vi "LS One Hour Data Loop.vi"(11 "FPGA OneHour Ref":T1) -> ()   [LabVIEW 2019]
uses:
  <vilib>/rvi/interface/nirviReadWriteControl/nirviReadWriteControl.xnode
  <vilib>/rvi/interface/nirviMethod/nirviMethod.xnode
  <vilib>/FPGAPlugInAG/sbRIO-9626/niLvFpga_ReadFifo_sbRIO-9626.vi
  <vilib>/rvi/errors/niLvFpgaMergeErrorWithErrorCode.vi
  FPGA Bitfiles/LSDurabilityMain_Alternate.lvbitx
  Controls/FPGA_OneHour_Reference.ctl
  NiFpgaLv.dll
  <vilib>/Utility/error.llb/Error Cluster From Error Code.vi
  <vilib>/rvi/errors/niLvFpgaAdjustHostInterfaceError.vi
panel:
  in  "LoopWait(ms)":u32=100
  in  "Sections":i32=100
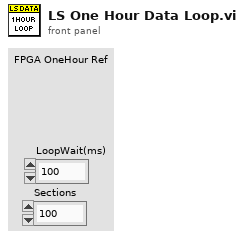
[diagram p1: front panel]
types:
  T1 = typedef "FPGA_OneHour_Reference.ctl" = refnum<k20>
  T2 = cluster{"FPGA OneHour Ref":T1, "Time":dbl, "PtsTaken":i32, "Pts/File":i32, "10AveWait":u32, "Stored Filepath":path, "FileIndex":i32, "FilesUsed":i32}
  T3 = enum16{"open", "replace", "create", "open or create", "replace or create", "replace or create with confirmation"}
  T4 = cluster{"Running?":bool, "Profile Record":bool, "RecordInterval":i32, "RecordDuration":i32, "RecordFreq":i32, "Data Filepath":path, "Hr Record":bool, "Serial Numbers":string[]}
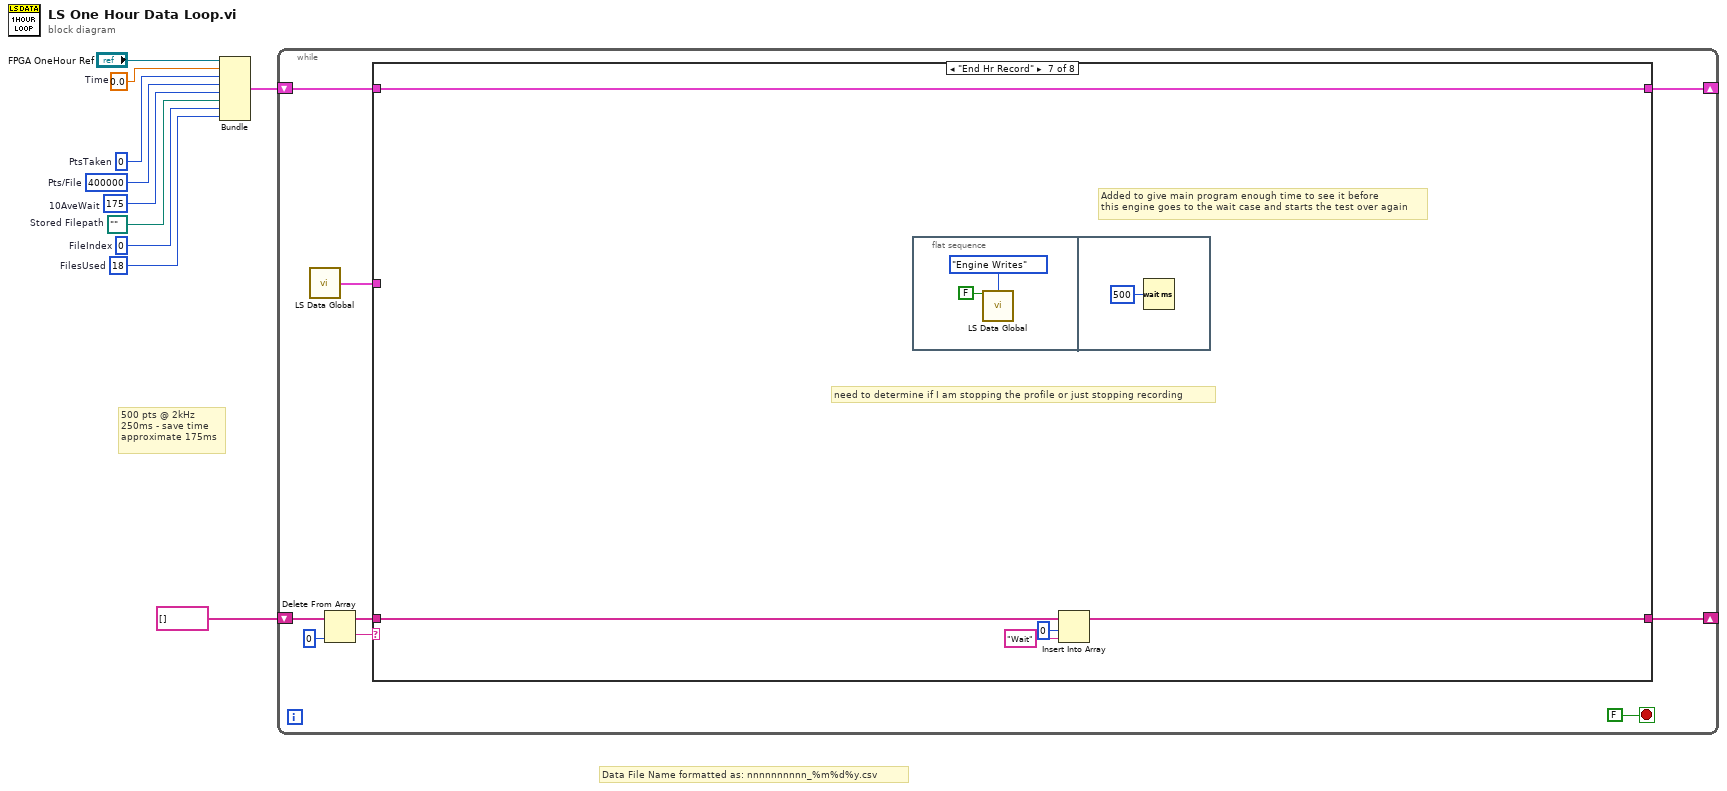
[diagram p0: block diagram]
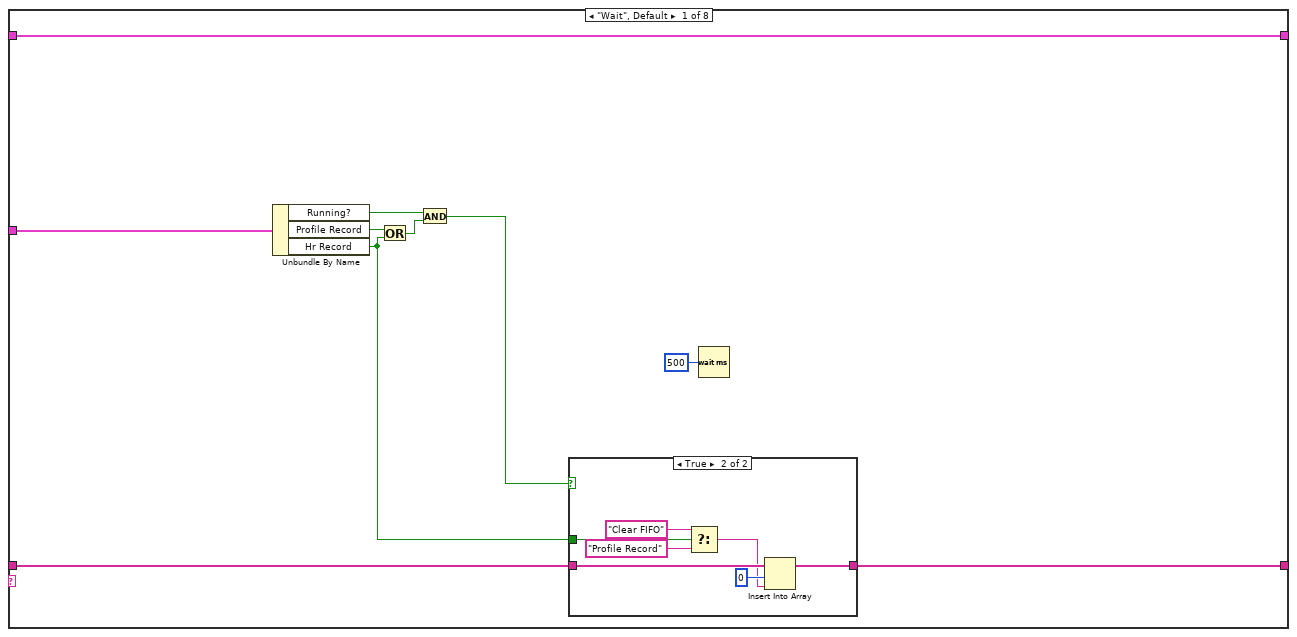
[diagram p2: hidden frame]
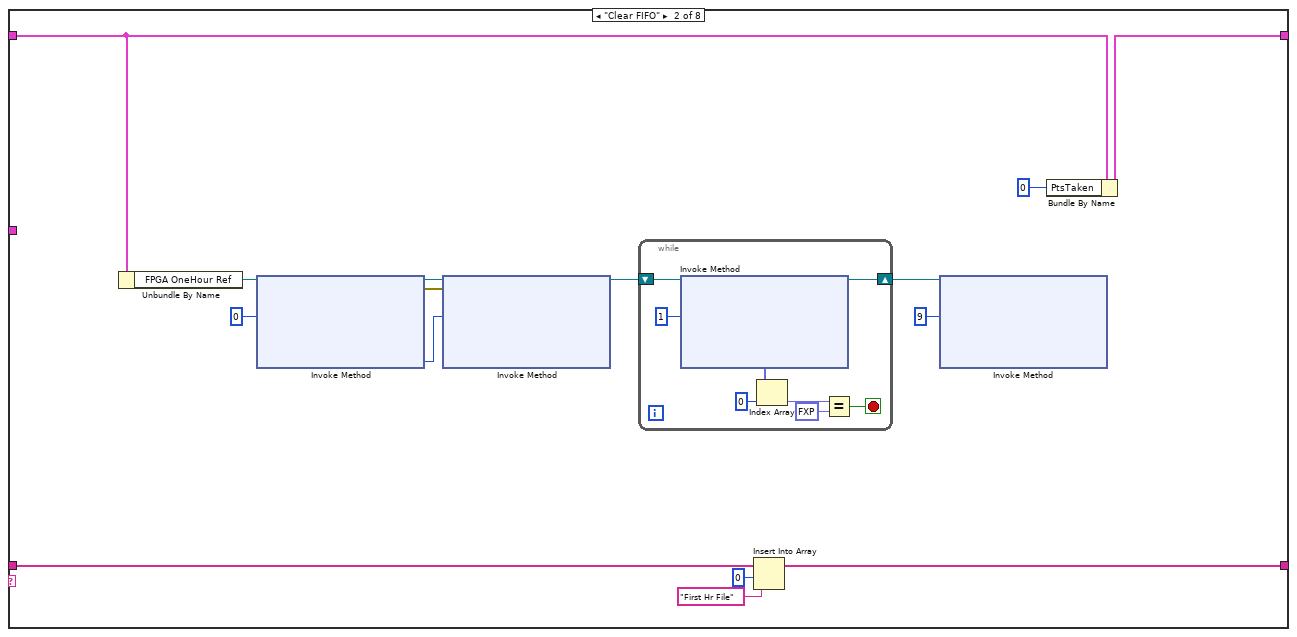
[diagram p4: hidden frame]
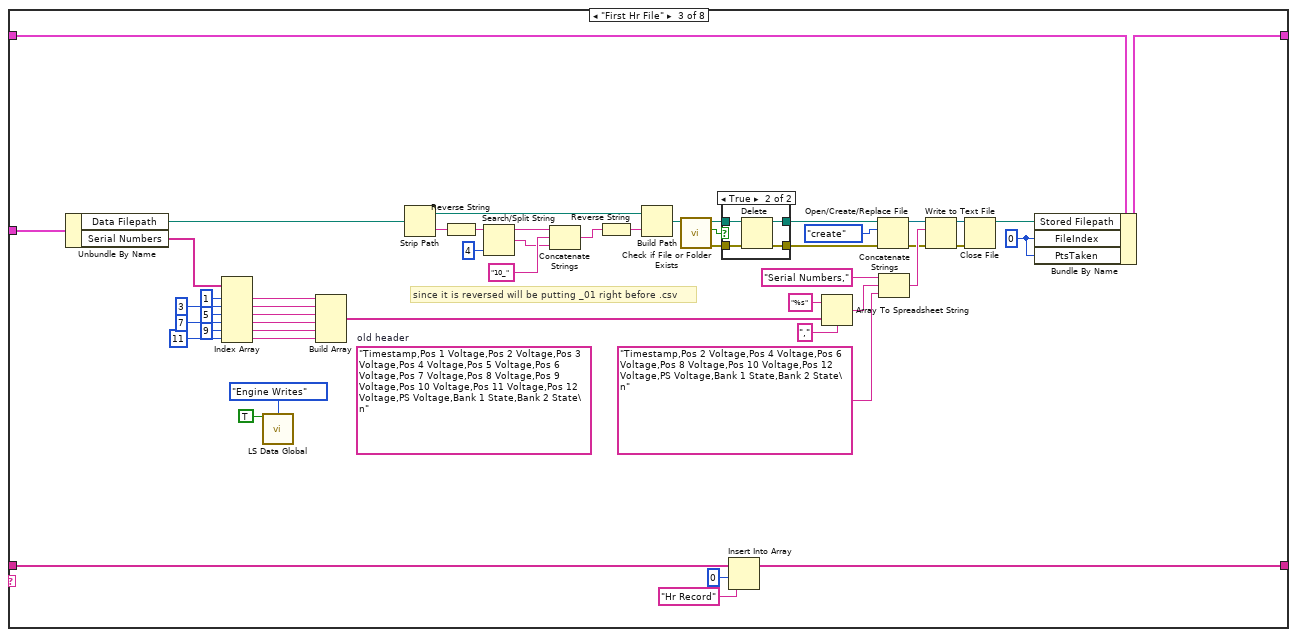
[diagram p5: hidden frame]
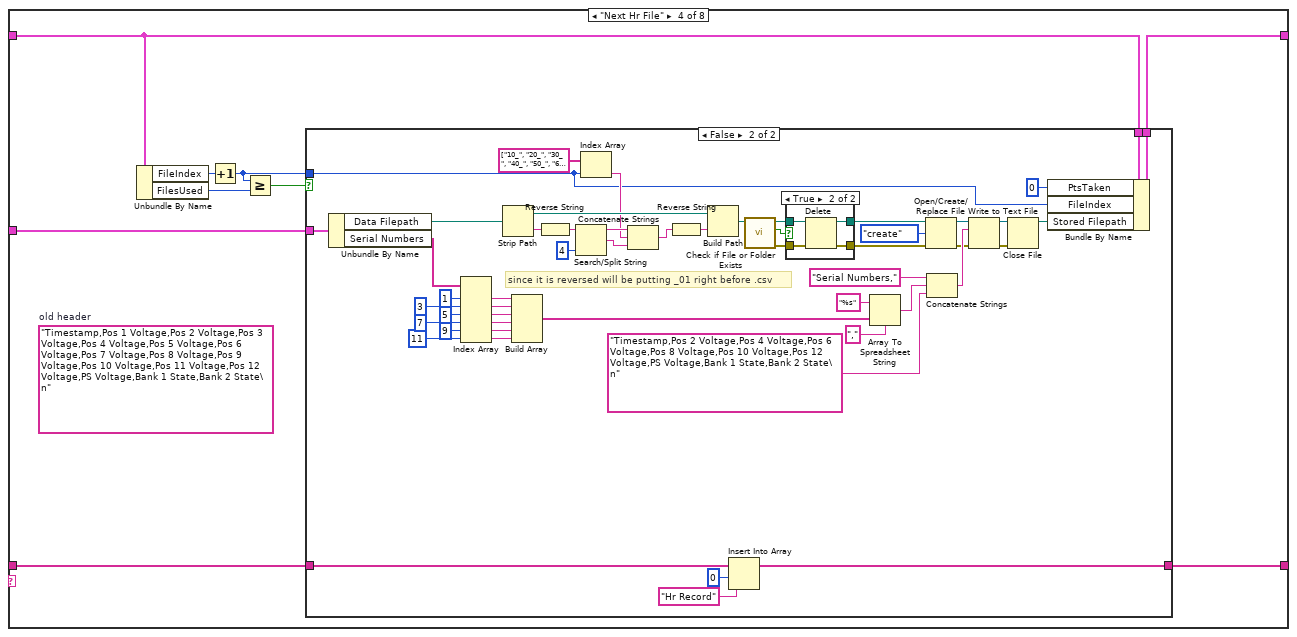
[diagram p7: hidden frame]
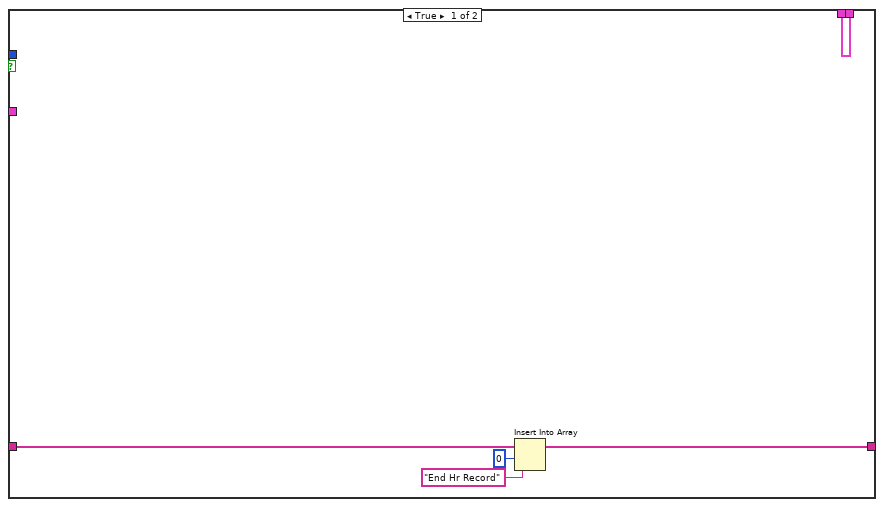
[diagram p8: hidden frame]
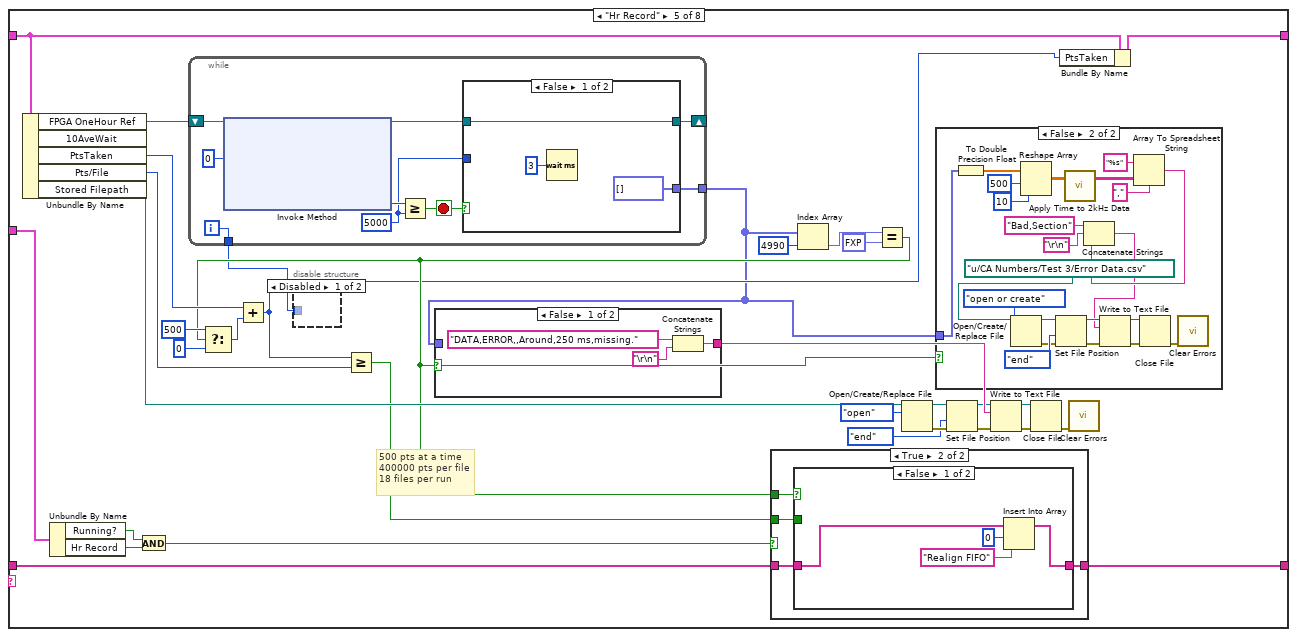
[diagram p10: hidden frame]
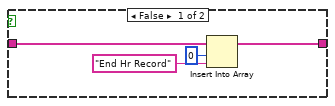
[diagram p13: hidden frame]
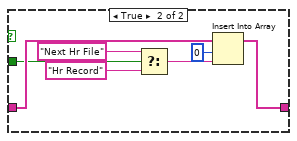
[diagram p14: hidden frame]
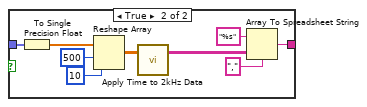
[diagram p15: hidden frame]
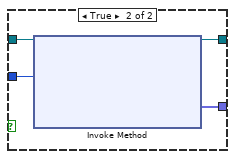
[diagram p16: hidden frame]
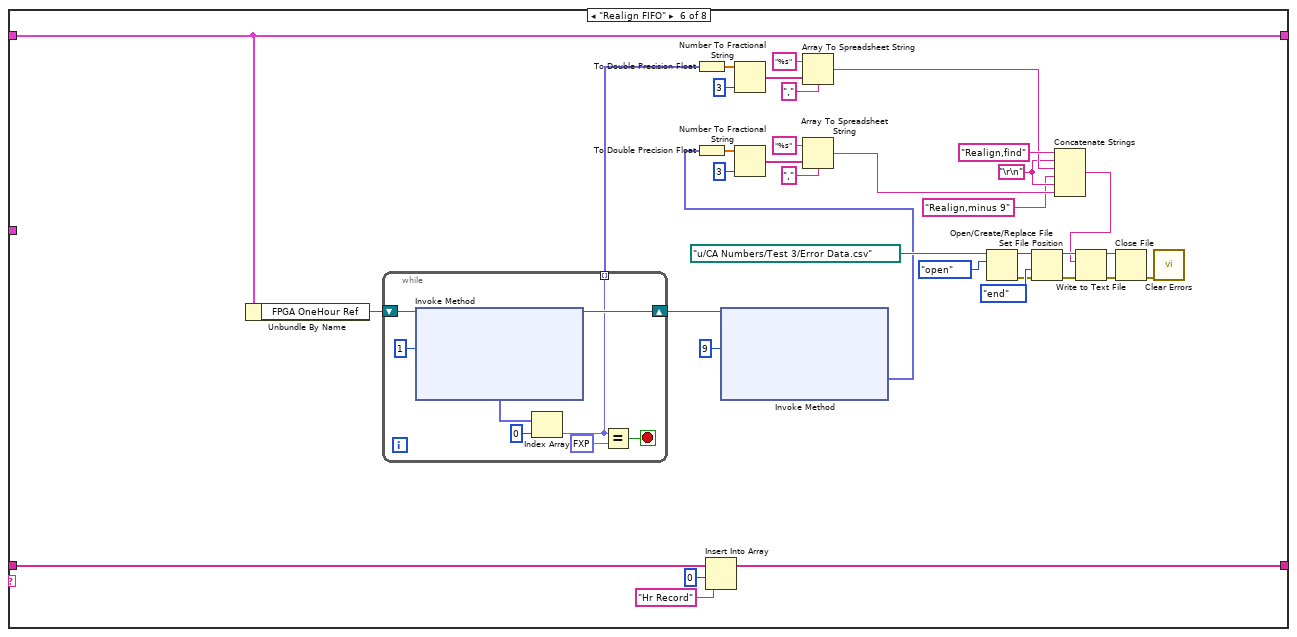
[diagram p17: hidden frame]
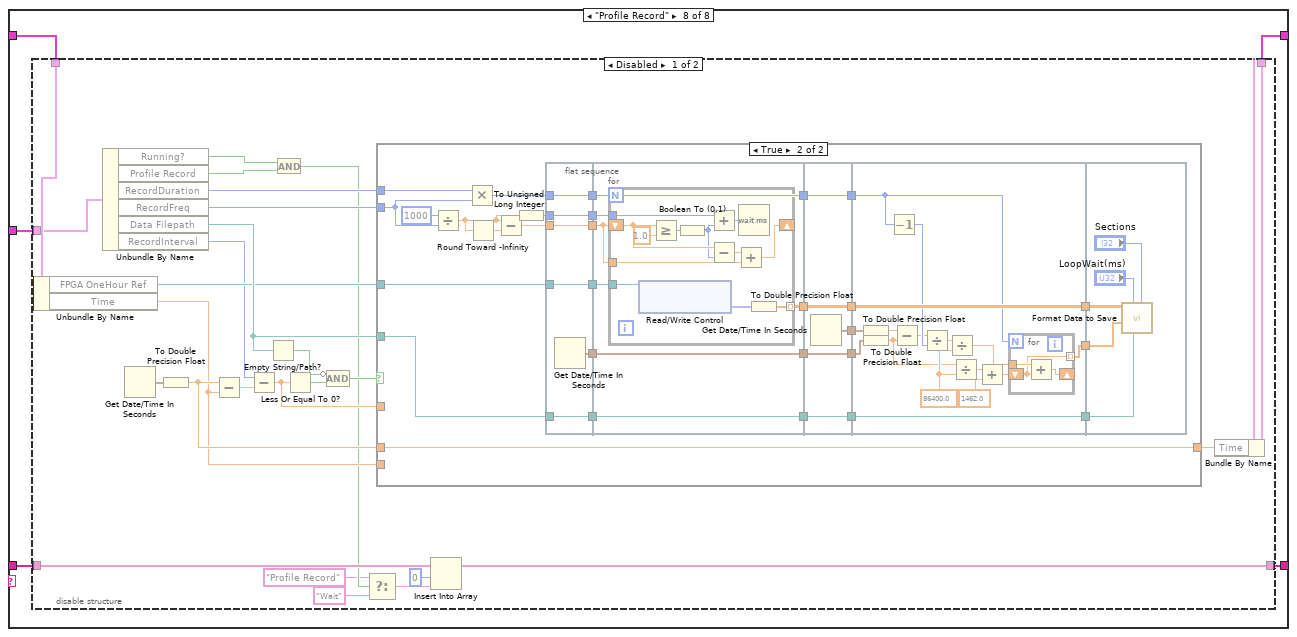
[diagram p18: hidden frame]
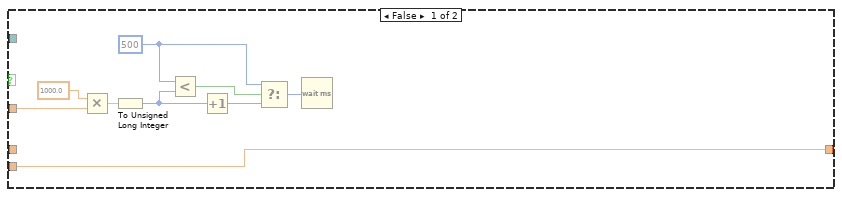
[diagram p19: hidden frame]
diagram:
  w1 = 18  # FilesUsed
  w2 = 400000  # Pts/File
  w4 = 0  # FileIndex
  w5 = path ""  # Stored Filepath
  w6 = u32 175  # 10AveWait
  w7 = 0  # PtsTaken
  w10 = 0.0  # Time
  # "500 pts @ 2kHz\n250ms - save time\napproximate 175ms"
  # "Data File Name formatted as: nnnnnnnnnn_%m%d%y.csv"
  n1 = Bundle("FPGA OneHour Ref"="FPGA OneHour Ref", "Time"=w10, "PtsTaken"=w7, "Pts/File"=w2, "10AveWait"=w6, "Stored Filepath"=w5, "FileIndex"=w4, "FilesUsed"=w1) -> (w9:T2)  [unwired: 1 in]
  n2 = while {
    shift-right: [w17] -> _
    shift-left: w9 -> [w18]
    shift-right: [w14] -> _
    shift-left: string[] [] -> [w16]
    stop <- FALSE stop-if-true
    n3 = call "LS Data Global.vi"() -> ("LS Cluster Out"=w15:T4)  [unwired: 12 in, 3 out]
    n4 = Delete From Array(array=w16, index=0) -> (deleted portion=w12:string, array with subset deleted=w11:string[])  [unwired: 1 in]
    n5 = case shown="\"End Hr Record\"" w12 {
      tunnel: w11 -> [w26 w47 w99 w119 w204 w322 w340 w346]
      tunnel: [w25 w45 w98 w125 w205 w321 w339 w345] -> w14
      tunnel: w15 -> [w27 _ w111 w127 w221 _ _ w347]
      tunnel: w18 -> [w24 w43 w112 w124 w199 w325 w341 w349]
      tunnel: [w24 w42 w110 w126 w198 w325 w341 w348] -> w17
      frame "Wait", Default {
        n6 = Unbundle By Name(w27) -> ("Running?"=w28:bool, "Profile Record"=w23:bool, "Hr Record"=w21:bool)
        n7 = Or(x=w23, y=w21) -> (x .or. y?=w22:bool)
        n8 = And(x=w28, y=w22) -> (x .and. y?=w20:bool)
        n9 = case shown="True" w20 {
          tunnel: w26 -> [w30 w37]
          tunnel: [w30 w36] -> w25
          tunnel: w21 -> [_ w34]
          frame False {
          }
          frame True {
            n10 = Select(t="Clear FIFO" ("new element/subarray"), s=w34, f="Profile Record" ("new element/subarray")) -> (s? t:f=w32:string)
            n11 = Insert Into Array(array=w37, index=0, new element=w32) -> (w36:string[])
          }
        }
        n12 = Wait (ms)(milliseconds to wait=u32 500) -> ()  [unwired: 1 out]
      }
      frame "Clear FIFO" {
        n13 = Unbundle By Name(w43) -> ("FPGA OneHour Ref"=w52:T1)
        n14 = xnode "Invoke Method"("FPGA VI Reference In"=w52, "Number of Elements"=u32 0) -> ("FPGA VI Reference Out"=w51:T1, "error out"=w50:errorcluster, "Elements Remaining"=w48:u32)  [unwired: 2 in, 1 out]
        n15 = xnode "Invoke Method"("FPGA VI Reference In"=w51, "error in"=w50, "Number of Elements"=w48) -> ("FPGA VI Reference Out"=w40:T1)  [unwired: 1 in, 3 out]
        n16 = while {
          shift-right: [w59] -> w38
          shift-left: w40 -> [w60]
          stop <- w53 stop-if-true
          n17 = xnode "Invoke Method"("FPGA VI Reference In"=w60, "Number of Elements"=u32 1) -> ("FPGA VI Reference Out"=w59:T1, "Data"=w57:fxp<+/-,18,5>[])  [unwired: 2 in, 2 out]
          n18 = Index Array(array=w57, index=0) -> (element=w55:fxp<+/-,18,5>)
          n19 = Equal?(x=w55, y=fxp<+/-,18,5> -15.0 ("lower limit")) -> (x = y?=w53:bool)
        }
        n20 = Insert Into Array(array=w47, index=0, new element="First Hr File" ("new element/subarray")) -> (w45:string[])
        n21 = xnode "Invoke Method"("FPGA VI Reference In"=w38, "Number of Elements"=u32 9) -> ()  [unwired: 2 in, 4 out]
        n22 = Bundle By Name(cluster=w43, "PtsTaken"=0) -> (w42:T2)
      }
      frame "First Hr File" {
        (unwired) "Timestamp,Pos 1 Voltage,Pos 2 Voltage,Pos 3 Voltage,Pos 4 Voltage,Pos 5 Voltage,Pos 6 Voltage,Pos 7 Voltage,Pos 8 Voltage,Pos 9 Voltage,Pos 10 Voltage,Pos 11 Voltage,Pos 12 Voltage,PS Voltage,Bank 1 State,Bank 2 State\n"  # old header
        w77 = 0 ("FileIndex")
        # "since it is reversed will be putting _01 right before .csv"
        n23 = Unbundle By Name(w111) -> ("Data Filepath"=w109:path, "Serial Numbers"=w62:string[])
        n24 = Index Array(array=w62, index #1=1 ("index"), index #2=3 ("index"), index #3=5 ("index"), index #4=7 ("index"), index #5=9 ("index"), index #6=11 ("index")) -> (element #1=w68:string, element #2=w67:string, element #3=w66:string, element #4=w65:string, element #5=w63:string, element #6=w64:string)
        n25 = call "LS Data Global.vi"("Recording In"=TRUE, "Mode"=enum16{"Read", "Engine Writes", "Main Writes"}."Engine Writes") -> ()  [unwired: 10 in, 4 out]
        n26 = Build Array(w68, w67, w66, w65, w63, w64) -> (w61:string[])
        n27 = Strip Path(path=w109) -> (stripped path=w108:path, name=w107:string)
        n28 = Reverse String(1:w107) -> (0:w105:string)
        n29 = Search/Split String(string=w105, offset (0)=4) -> (substring before match=w103:string, match + rest of string=w100:string)  [unwired: 1 in, 1 out]
        n30 = Concatenate Strings(w103, "10_", w100) -> (w102:string)
        n31 = Reverse String(1:w102) -> (0:w106:string)
        n32 = Build Path(base path=w108, name or relative path=w106) -> (appended path=w95:path)
        n33 = call <vilib>:"Check if File or Folder Exists.vi"("path"=w95) -> ("error out"=w80:errorcluster, "file or folder exists?"=w94:bool, "dup path"=w93:path)  [unwired: 8 in]
        n34 = case shown="True" w94 {
          tunnel: w93 -> [w114 w118]
          tunnel: [w114 w117] -> w82
          tunnel: w80 -> [w113 w116]
          tunnel: [w113 w115] -> w79
          frame False {
          }
          frame True {
            n35 = Delete(path (use dialog)=w118, error in=w116) -> (deleted path=w117:path, error out=w115:errorcluster)  [unwired: 3 in, 1 out]
          }
        }
        n36 = Insert Into Array(array=w99, index=0, new element="Hr Record" ("new element/subarray")) -> (w98:string[])
        n37 = Array To Spreadsheet String(delimiter (Tab)=",", array=w61, 3:"%s" ("format string")) -> (spreadsheet string=w92:string)
        n38 = Open/Create/Replace File(file path (use dialog)=w82, error in=w79, operation (0:open)=T3."create") -> (refnum out=w86:refnum<file>, error out=w84:errorcluster)  [unwired: 3 in, 1 out]
        n39 = Concatenate Strings("Serial Numbers," ("string"), w92, "Timestamp,Pos 2 Voltage,Pos 4 Voltage,Pos 6 Voltage,Pos 8 Voltage,Pos 10 Voltage,Pos 12 Voltage,PS Voltage,Bank 1 State,Bank 2 State\n") -> (w89:string)
        n40 = Write to Text File(file (use dialog)=w86, text=w89, error in=w84) -> (refnum out=w87:refnum<file>, error out=w85:errorcluster)  [unwired: 1 in, 1 out]
        n41 = Close File(refnum=w87, error in=w85) -> (path=w81:path)  [unwired: 1 out]
        n42 = Bundle By Name(cluster=w112, "Stored Filepath"=w81, "FileIndex"=w77, "PtsTaken"=w77) -> (w110:T2)
      }
      frame "Next Hr File" {
        (unwired) "Timestamp,Pos 1 Voltage,Pos 2 Voltage,Pos 3 Voltage,Pos 4 Voltage,Pos 5 Voltage,Pos 6 Voltage,Pos 7 Voltage,Pos 8 Voltage,Pos 9 Voltage,Pos 10 Voltage,Pos 11 Voltage,Pos 12 Voltage,PS Voltage,Bank 1 State,Bank 2 State\n"  # old header
        n43 = Unbundle By Name(w124) -> ("FileIndex"=w123:i32, "FilesUsed"=w122:i32)
        n44 = Increment(x=w123) -> (x+1=w121:i32)
        n45 = Greater Or Equal?(x=w121, y=w122) -> (x >= y?=w120:bool)
        n46 = case shown="False" w120 {
          tunnel: w127 -> [_ w184]
          tunnel: [w132 w183] -> w126
          tunnel: [w130 w172] -> w125
          tunnel: w124 -> [w132 w152]
          tunnel: w121 -> [_ w149]
          tunnel: w119 -> [w131 w173]
          frame True {
            n47 = Insert Into Array(array=w131, index=0, new element="End Hr Record" ("new element/subarray")) -> (w130:string[])
          }
          frame False {
            # "since it is reversed will be putting _01 right before .csv"
            n48 = Unbundle By Name(w184) -> ("Data Filepath"=w182:path, "Serial Numbers"=w134:string[])
            n49 = Index Array(array=w134, index #1=1 ("index"), index #2=3 ("index"), index #3=5 ("index"), index #4=7 ("index"), index #5=9 ("index"), index #6=11 ("index")) -> (element #1=w140:string, element #2=w139:string, element #3=w138:string, element #4=w137:string, element #5=w135:string, element #6=w136:string)
            n50 = Strip Path(path=w182) -> (stripped path=w181:path, name=w180:string)
            n51 = Build Array(w140, w139, w138, w137, w135, w136) -> (w133:string[])
            n52 = Reverse String(1:w180) -> (0:w178:string)
            n53 = Search/Split String(string=w178, offset (0)=4) -> (substring before match=w176:string, match + rest of string=w174:string)  [unwired: 1 in, 1 out]
            n54 = Index Array(array=string[] ["10_", "20_", "30_", "40_", "50_", "60_", "70_", "80_", "90_", "01_", "11_", "21_", "31_", "41_", "51_", "61_", "71_", "81_", "91_", "02_", "12_", "22_", "32_", "42_", "52_", "62_", "72_", "82_", "92_", "03_", "13_", "23_"], index=w149) -> (element=w150:string)
            n55 = Concatenate Strings(w176, w150, w174) -> (w175:string)
            n56 = Reverse String(1:w175) -> (0:w179:string)
            n57 = Build Path(base path=w181, name or relative path=w179) -> (appended path=w169:path)
            n58 = Insert Into Array(array=w173, index=0, new element="Hr Record" ("new element/subarray")) -> (w172:string[])
            n59 = call <vilib>:"Check if File or Folder Exists.vi"("path"=w169) -> ("error out"=w154:errorcluster, "file or folder exists?"=w168:bool, "dup path"=w167:path)  [unwired: 8 in]
            n60 = case shown="True" w168 {
              tunnel: w167 -> [w186 w190]
              tunnel: [w186 w189] -> w156
              tunnel: w154 -> [w185 w188]
              tunnel: [w185 w187] -> w153
              frame False {
              }
              frame True {
                n61 = Delete(path (use dialog)=w190, error in=w188) -> (deleted path=w189:path, error out=w187:errorcluster)  [unwired: 3 in, 1 out]
              }
            }
            n62 = Array To Spreadsheet String(delimiter (Tab)=",", array=w133, 3:"%s" ("format string")) -> (spreadsheet string=w166:string)
            n63 = Open/Create/Replace File(file path (use dialog)=w156, error in=w153, operation (0:open)=T3."create") -> (refnum out=w160:refnum<file>, error out=w158:errorcluster)  [unwired: 3 in, 1 out]
            n64 = Concatenate Strings("Serial Numbers," ("string"), w166, "Timestamp,Pos 2 Voltage,Pos 4 Voltage,Pos 6 Voltage,Pos 8 Voltage,Pos 10 Voltage,Pos 12 Voltage,PS Voltage,Bank 1 State,Bank 2 State\n") -> (w163:string)
            n65 = Write to Text File(file (use dialog)=w160, text=w163, error in=w158) -> (refnum out=w161:refnum<file>, error out=w159:errorcluster)  [unwired: 1 in, 1 out]
            n66 = Close File(refnum=w161, error in=w159) -> (path=w155:path)  [unwired: 1 out]
            n67 = Bundle By Name(cluster=w152, "PtsTaken"=0, "FileIndex"=w149, "Stored Filepath"=w155) -> (w183:T2)
          }
        }
      }
      frame "Hr Record" {
        # "500 pts at a time\n400000 pts per file\n18 files per run"
        n68 = Unbundle By Name(w199) -> ("FPGA OneHour Ref"=w193:T1, "PtsTaken"=w203:i32, "Pts/File"=w197:i32, "Stored Filepath"=w210:path)  [unwired: 1 out]
        n69 = Unbundle By Name(w221) -> ("Running?"=w222:bool, "Hr Record"=w223:bool)
        n70 = And(x=w222, y=w223) -> (x .and. y?=w206:bool)
        n71 = while {
          shift-right: [w280] -> _
          shift-left: w193 -> [w283]
          tunnel: [w279] -> w192
          tunnel: [w277] -> w191
          i -> [w277]
          stop <- w278 stop-if-true
          w282 = u32 5000 ("y")
          n72 = xnode "Invoke Method"("FPGA VI Reference In"=w283, "Number of Elements"=u32 0) -> ("FPGA VI Reference Out"=w281:T1, "Elements Remaining"=w284:u32)  [unwired: 2 in, 2 out]
          n73 = Greater Or Equal?(x=w284, y=w282) -> (x >= y?=w278:bool)
          n74 = case shown="False" w278 {
            tunnel: w282 -> [_ w292]
            tunnel: w281 -> [w288 w291]
            tunnel: [w288 w290] -> w280
            tunnel: [fxp<+/-,18,5>[] [] ("Data") w289] -> w279
            frame False {
              n75 = Wait (ms)(milliseconds to wait=u32 3) -> ()  [unwired: 1 out]
            }
            frame True {
              n76 = xnode "Invoke Method"("FPGA VI Reference In"=w291, "Number of Elements"=w292) -> ("FPGA VI Reference Out"=w290:T1, "Data"=w289:fxp<+/-,18,5>[])  [unwired: 2 in, 2 out]
            }
          }
        }
        n77 = disable-structure shown="Disabled" {
          disable-tunnel: w191 -> [_ _]
          frame Disabled {
          }
          frame Enabled {
          }
        }
        n78 = Index Array(array=w192, index=4990) -> (element=w208:fxp<+/-,18,5>)
        n79 = Equal?(x=w208, y=fxp<+/-,18,5> -15.0) -> (x = y?=w195:bool)
        n80 = Select(t=500 ("PtsTaken"), s=w195, f=0 ("PtsTaken")) -> (s? t:f=w200:i32)
        n81 = Add(x=w203, y=w200) -> (x+y=w194:i32)
        n82 = Greater Or Equal?(x=w194, y=w197) -> (x >= y?=w196:bool)
        n83 = case shown="False" w195 {
          tunnel: [w265 w272] -> w213
          tunnel: w192 -> [_ w269]
          frame False {
            n84 = Concatenate Strings("DATA,ERROR,,Around,250 ms,missing." ("string"), "\r\n") -> (w265:string)
          }
          frame True {
            n85 = To Single Precision Float(number=w269) -> (single precision float=w268:sgl[])
            n86 = Reshape Array(w268, 500 ("dimension size"), 10 ("dimension size")) -> (w271:sgl[][])
            n87 = call "Apply Time to 2kHz Data.vi"("Data In"=w271) -> ("Data Out"=w270:string[][])  [unwired: 2 in]
            n88 = Array To Spreadsheet String(delimiter (Tab)=",", array=w270, 3:"%s" ("format string")) -> (spreadsheet string=w272:string)
          }
        }
        n89 = case shown="True" w206 {
          tunnel: w204 -> [w248 w252]
          tunnel: [w247 w251] -> w205
          tunnel: w195 -> [_ w253]
          tunnel: w196 -> [_ w250]
          frame False {
            n90 = Insert Into Array(array=w248, index=0, new element="End Hr Record") -> (w247:string[])
          }
          frame True {
            n91 = case shown="False" w253 {
              tunnel: w252 -> [w257 w264]
              tunnel: [w256 w263] -> w251
              tunnel: w250 -> [_ w261]
              frame False {
                n92 = Insert Into Array(array=w257, index=0, new element="Realign FIFO" ("new element/subarray")) -> (w256:string[])
              }
              frame True {
                n93 = Select(t="Next Hr File", s=w261, f="Hr Record") -> (s? t:f=w260:string)
                n94 = Insert Into Array(array=w264, index=0, new element=w260) -> (w263:string[])
              }
            }
          }
        }
        n95 = Open/Create/Replace File(file path (use dialog)=w210, operation (0:open)=T3."open") -> (refnum out=w216:refnum<file>, error out=w215:errorcluster)  [unwired: 4 in, 1 out]
        n96 = case shown="False" w195 {
          tunnel: w192 -> [_ w240]
          frame True {
          }
          frame False {
            n97 = To Double Precision Float(number=w240) -> (double precision float=w243:dbl[])
            n98 = Open/Create/Replace File(file path (use dialog)=path "u:/CA Numbers/Test 3/Error Data.csv" ("base path"), operation (0:open)=T3."open or create") -> (refnum out=w233:refnum<file>, error out=w234:errorcluster)  [unwired: 4 in, 1 out]
            n99 = Reshape Array(w243, 500 ("dimension size"), 10 ("dimension size")) -> (w239:dbl[][])
            n100 = Set File Position(refnum=w233, from (0:start)=enum16{"start", "end", "current"}."end", error in=w234) -> (refnum out=w236:refnum<file>, error out=w237:errorcluster)  [unwired: 1 in]
            n101 = call "Apply Time to 2kHz Data.vi"("Data In"=w239) -> ("Data Out"=w238:string[][])  [unwired: 2 in]
            n102 = Array To Spreadsheet String(delimiter (Tab)=",", array=w238, 3:"%s" ("format string")) -> (spreadsheet string=w226:string)
            n103 = Concatenate Strings("Bad,Section" ("string"), "\r\n", w226) -> (w225:string)
            n104 = Write to Text File(file (use dialog)=w236, text=w225, error in=w237) -> (refnum out=w230:refnum<file>, error out=w229:errorcluster)  [unwired: 1 in, 1 out]
            n105 = Close File(refnum=w230, error in=w229) -> (error out=w231:errorcluster)  [unwired: 1 out]
            n106 = call <vilib>:"Clear Errors.vi"("error in (no error)"=w231) -> ()  [unwired: 5 in, 2 out]
          }
        }
        n107 = Set File Position(refnum=w216, from (0:start)=enum16{"start", "end", "current"}."end", error in=w215) -> (refnum out=w212:refnum<file>, error out=w211:errorcluster)  [unwired: 1 in]
        n108 = Write to Text File(file (use dialog)=w212, text=w213, error in=w211) -> (refnum out=w219:refnum<file>, error out=w220:errorcluster)  [unwired: 1 in, 1 out]
        n109 = Close File(refnum=w219, error in=w220) -> (error out=w218:errorcluster)  [unwired: 1 out]
        n110 = Bundle By Name(cluster=w199, "PtsTaken"=w194) -> (w198:T2)
        n111 = call <vilib>:"Clear Errors.vi"("error in (no error)"=w218) -> ()  [unwired: 5 in, 2 out]
      }
      frame "Realign FIFO" {
        w301 = "\r\n"
        n112 = Unbundle By Name(w325) -> ("FPGA OneHour Ref"=w328:T1)
        n113 = while {
          shift-right: [w335] -> w326
          shift-left: w328 -> [w336]
          tunnel: [w329] -> w305 mode=indexing
          stop <- w330 stop-if-true
          n114 = xnode "Invoke Method"("FPGA VI Reference In"=w336, "Number of Elements"=u32 1) -> ("FPGA VI Reference Out"=w335:T1, "Data"=w333:fxp<+/-,18,5>[])  [unwired: 2 in, 2 out]
          n115 = Index Array(array=w333, index=0) -> (element=w329:fxp<+/-,18,5>)
          n116 = Equal?(x=w329, y=fxp<+/-,18,5> -15.0 ("lower limit")) -> (x = y?=w330:bool)
        }
        n117 = To Double Precision Float(number=w305) -> (double precision float=w303:dbl[])
        n118 = Insert Into Array(array=w322, index=0, new element="Hr Record" ("new element/subarray")) -> (w321:string[])
        n119 = xnode "Invoke Method"("FPGA VI Reference In"=w326, "Number of Elements"=u32 9) -> ("Data"=w295:fxp<+/-,18,5>[])  [unwired: 2 in, 3 out]
        n120 = To Double Precision Float(number=w295) -> (double precision float=w299:dbl[])
        n121 = Number To Fractional String(number=w303, precision (6)=i16 3) -> (F-format string=w302:string[])  [unwired: 2 in]
        n122 = Number To Fractional String(number=w299, precision (6)=i16 3) -> (F-format string=w300:string[])  [unwired: 2 in]
        n123 = Array To Spreadsheet String(delimiter (Tab)=",", array=w302, 3:"%s" ("format string")) -> (spreadsheet string=w308:string)
        n124 = Array To Spreadsheet String(delimiter (Tab)=",", array=w300, 3:"%s" ("format string")) -> (spreadsheet string=w294:string)
        n125 = Open/Create/Replace File(file path (use dialog)=path "u:/CA Numbers/Test 3/Error Data.csv" ("base path"), operation (0:open)=T3."open") -> (refnum out=w314:refnum<file>, error out=w315:errorcluster)  [unwired: 4 in, 1 out]
        n126 = Set File Position(refnum=w314, from (0:start)=enum16{"start", "end", "current"}."end", error in=w315) -> (refnum out=w317:refnum<file>, error out=w318:errorcluster)  [unwired: 1 in]
        n127 = Concatenate Strings("Realign,find" ("string"), w301, w308, "Realign,minus 9" ("string"), w301, w294) -> (w307:string)
        n128 = Write to Text File(file (use dialog)=w317, text=w307, error in=w318) -> (refnum out=w311:refnum<file>, error out=w310:errorcluster)  [unwired: 1 in, 1 out]
        n129 = Close File(refnum=w311, error in=w310) -> (error out=w312:errorcluster)  [unwired: 1 out]
        n130 = call <vilib>:"Clear Errors.vi"("error in (no error)"=w312) -> ()  [unwired: 5 in, 2 out]
      }
      frame "End Hr Record" {
        # "Added to give main program enough time to see it before\nthis engine goes to the wait case and starts the test over again"
        # "need to determine if I am stopping the profile or just stopping recording"
        n131 = flat-sequence {
          frame #0 {
            n132 = call "LS Data Global.vi"("Recording In"=FALSE, "Mode"=enum16{"Read", "Engine Writes", "Main Writes"}."Engine Writes") -> ()  [unwired: 10 in, 4 out]
          }
          frame #1 {
            n133 = Wait (ms)(milliseconds to wait=u32 500) -> ()  [unwired: 1 out]
          }
        }
        n134 = Insert Into Array(array=w340, index=0, new element="Wait" ("new element/subarray")) -> (w339:string[])
      }
      frame "Profile Record" {
        n135 = disable-structure shown="Disabled" {
          disable-tunnel: w349 -> [w375 w469]
          disable-tunnel: [w374 w469] -> w348
          disable-tunnel: w347 -> [w373 _]
          disable-tunnel: w346 -> [w356 w468]
          disable-tunnel: [w355 w468] -> w345
          frame Disabled {
            n136 = Unbundle By Name(w375) -> ("FPGA OneHour Ref"=w367:T1, "Time"=w361:dbl)
            n137 = Unbundle By Name(w373) -> ("Running?"=w358:bool, "Profile Record"=w357:bool, "RecordDuration"=w370:i32, "RecordFreq"=w371:i32, "Data Filepath"=w372:path, "RecordInterval"=w359:i32)
            n138 = Get Date/Time In Seconds() -> (seconds since 1Jan1904=w369:timestamp)
            n139 = To Double Precision Float(number=w369) -> (double precision float=w362:dbl)
            n140 = Subtract(x=w362, y=w361) -> (x-y=w366:dbl)
            n141 = Subtract(x=w359, y=w366) -> (x-y=w360:dbl)
            n142 = Empty String/Path?(string/path=w372) -> (empty?=w364:bool)
            n143 = And(x=w358, y=w357) -> (x .and. y?=w353:bool)
            n144 = Less Or Equal To 0?(x=w360) -> (x <= 0?=w365:bool)
            n145 = Compound Arithmetic op=AND(invert w364, w365) -> (w363:bool)
            n146 = Select(t="Profile Record", s=w353, f="Wait") -> (s? t:f=w350:string)
            n147 = case shown="True" w363 {
              tunnel: w371 -> [_ w406]
              tunnel: w370 -> [_ w412]
              tunnel: w367 -> [_ w409]
              tunnel: w362 -> [_ w408]
              tunnel: [w384 w408] -> w368
              tunnel: w361 -> [w384 _]
              tunnel: w360 -> [w378 _]
              tunnel: w372 -> [_ w385]
              frame False {
                w383 = u32 500 ("milliseconds to wait")
                n148 = Multiply(x=1000.0 ("y"), y=w378) -> (x*y=w380:dbl)
                n149 = To Unsigned Long Integer(number=w380) -> (unsigned 32bit integer=w377:u32)
                n150 = Less?(x=w383, y=w377) -> (x < y?=w381:bool)
                n151 = Increment(x=w377) -> (x+1=w376:u32)
                n152 = Select(t=w383, s=w381, f=w376) -> (s? t:f=w382:u32)
                n153 = Wait (ms)(milliseconds to wait=w382) -> ()  [unwired: 1 out]
              }
              frame True {
                n154 = Divide(x=1000, y=w406) -> (x/y=w411:dbl)
                n155 = Multiply(x=w412, y=w406) -> (x*y=w399:i32)
                n156 = Round Toward -Infinity(1:w411) -> (0:w413:dbl)
                n157 = Subtract(x=w411, y=w413) -> (x-y=w405:dbl)
                n158 = To Unsigned Long Integer(number=w411) -> (unsigned 32bit integer=w410:u32)
                n159 = flat-sequence {
                  tunnel: w405 -> [w416]
                  tunnel: w409 -> [w417]
                  tunnel: w410 -> [w418]
                  tunnel: w399 -> [w419]
                  tunnel: [w419] -> w404
                  tunnel: [w418] -> w403
                  tunnel: [w417] -> w402
                  tunnel: [w416] -> w401
                  tunnel: [w415] -> w394
                  tunnel: [w414] -> w386
                  tunnel: w385 -> [w414]
                  tunnel: w404 -> [w422]
                  tunnel: w403 -> [w426]
                  tunnel: w402 -> [w425]
                  tunnel: w401 -> [w420]
                  tunnel: [w424] -> w400
                  tunnel: [w423] -> w395
                  tunnel: w394 -> [w423]
                  tunnel: [w422] -> w392
                  tunnel: [w421] -> w387
                  tunnel: w386 -> [w421]
                  tunnel: w400 -> [w443]
                  tunnel: [w443] -> w398
                  tunnel: [w442] -> w397
                  tunnel: [w441] -> w396
                  tunnel: w395 -> [w441]
                  tunnel: [w440] -> w393
                  tunnel: w392 -> [w440]
                  tunnel: [w439] -> w388
                  tunnel: w387 -> [w439]
                  tunnel: w398 -> [w459]
                  tunnel: w397 -> [w453]
                  tunnel: w396 -> [w452]
                  tunnel: w393 -> [w451]
                  tunnel: [w459] -> w391
                  tunnel: [w449] -> w390
                  tunnel: [w446] -> w389
                  tunnel: w388 -> [w446]
                  tunnel: w389 -> [w465]
                  tunnel: w390 -> [w466]
                  tunnel: w391 -> [w467]
                  frame #0 {
                    n160 = Get Date/Time In Seconds() -> (seconds since 1Jan1904=w415:timestamp)
                  }
                  frame #1 {
                    n161 = for {
                      N: w422 -> [_]
                      tunnel: w426 -> [w438]
                      shift-right: [w435] -> _
                      shift-left: w420 -> [w436]
                      tunnel: w420 -> [w434]
                      tunnel: w425 -> [w433]
                      tunnel: [w431] -> w424 mode=indexing
                      n162 = xnode "Read/Write Control"("FPGA VI Reference In"=w433) -> ("Analog Inputs"=w432:fxp<+/-,28,17>[])  [unwired: 1 in, 2 out]
                      n163 = Greater Or Equal?(x=w436, y=1.0) -> (x >= y?=w429:bool)
                      n164 = Boolean To (0,1)(Boolean=w429) -> (0, 1=w428:i16)
                      n165 = Add(x=w438, y=w428) -> (x+y=w437:u32)
                      n166 = Subtract(x=w436, y=w428) -> (x-y=w427:dbl)
                      n167 = Add(x=w427, y=w434) -> (x+y=w435:dbl)
                      n168 = Wait (ms)(milliseconds to wait=w437) -> ()  [unwired: 1 out]
                      n169 = To Double Precision Float(number=w432) -> (double precision float=w431:dbl[])
                    }
                  }
                  frame #2 {
                    n170 = Get Date/Time In Seconds() -> (seconds since 1Jan1904=w442:timestamp)
                  }
                  frame #3 {
                    w448 = 86400.0 ("y")
                    n171 = To Double Precision Float(number=w453) -> (double precision float=w447:dbl)
                    n172 = To Double Precision Float(number=w452) -> (double precision float=w444:dbl)
                    n173 = Decrement(x=w451) -> (x-1=w450:i32)
                    n174 = Subtract(x=w447, y=w444) -> (x-y=w445:dbl)
                    n175 = Divide(x=w445, y=w450) -> (x/y=w454:dbl)
                    n176 = Divide(x=w454, y=w448) -> (x/y=w458:dbl)
                    n177 = Divide(x=w444, y=w448) -> (x/y=w455:dbl)
                    n178 = Add(x=w455, y=1462.0) -> (x+y=w457:dbl)
                    n179 = for {
                      N: w451 -> [_]
                      shift-right: [w460] -> _
                      shift-left: w457 -> [w461]
                      tunnel: w458 -> [w462]
                      tunnel: [w461] -> w449 mode=indexing
                      n180 = Add(x=w462, y=w461) -> (x+y=w460:dbl)
                    }
                  }
                  frame #4 {
                    n181 = call "Format Data to Save.vi"("Sections"="Sections", "FilePath"=w465, "LoopBeginWait(ms)"="LoopWait(ms)", "Time"=w466, "Data"=w467) -> ()  [unwired: 7 in]
                  }
                }
              }
            }
            n182 = Insert Into Array(array=w356, index=0, new element=w350) -> (w355:string[])
            n183 = Bundle By Name(cluster=w375, "Time"=w368) -> (w374:T2)
          }
          frame Enabled {
          }
        }
      }
    }
  }
